vi "DeleteSubscriber.vi"(8 "ErrorIn":errorcluster, 9 "TraceQueue":refnum<queue>, 11 "TAFTraceWindowIn":refnum<class "TAFTraceWindow.lvclass">) -> (0 "ErrorOut":errorcluster, 3 "TAFTraceWindowOut":refnum<class "TAFTraceWindow.lvclass">)   [LabVIEW 2021, in "TAFTraceWindow.lvclass"]
uses:
  TAFTraceWindow.lvclass
  C:/Localdata/Projects/TriekselSoft/TriekselsoftApplicationFramework/Source/.Externals/Library_YAF/YActor/YActor.lvclass
  Library_YAF/YActor/YActor.lvclass/YActor.ctl
  Library_YAF/YActor/ExeCmd_sync.vi
  Library_YAF/YActor/private/SendCommand.vi
  Library_YAF/YActor/private/WaitForReply.vi
  Library_YAF/YActor/private/CreateLocalVI.vi
  Library_YAF/YActor/private/ExeuteInlineVI.vi
  Library_YAF/YActor/private/GetRemoteVIRef.vi
  Library_YAF/YActor/private/GetNameOfVI.vi
  Library_YAF/YActor/QuickCast.vi
  Library_YAF/YActor/private/VINameProperty.vi
  Library_YAF/YActor/private/MessageCounter.vi
  Library_YAF/YActor/InlineReferencePool.vi
  Library_YAF/YActor/private/ExecuteVI.vi
  Library_YAF/YActor/YActor.lvclass
  TAFTraceWindow.lvclass/TAFTraceWindow.ctl
  C:/Localdata/Projects/TriekselSoft/TriekselsoftApplicationFramework/Source/.Externals/Library_YAF/YAFTAF/YAFTAF.lvclass
  C:/Localdata/Projects/TriekselSoft/TriekselsoftApplicationFramework/Source/.Externals/Interface_UserInterface_IFrontPanel/IFrontPanel/IFrontPanel.lvclass
  C:/Localdata/Projects/TriekselSoft/TriekselsoftApplicationFramework/Source/IInterface/IInterface.lvclass
  C:/Localdata/Projects/TriekselSoft/TriekselsoftApplicationFramework/Source/.Externals/Interface_Object_ICreateDestroy/ICreateDestroy/ICreateDestroy.lvclass
  C:/Localdata/Projects/TriekselSoft/TriekselsoftApplicationFramework/Source/.Externals/Interface_Object_IPersistentData/IPersistentData/IPersistentData.lvclass
  C:/Localdata/Projects/TriekselSoft/TriekselsoftApplicationFramework/Source/.Externals/Interface_TAF_ITAFObject/ITAFObject/ITAFObject.lvclass
  C:/Localdata/Projects/TriekselSoft/TriekselsoftApplicationFramework/Source/.Externals/Library_TAF_TraceWindow/TAFTraceWindow/TAFTraceWindow.lvclass
  C:/Localdata/Projects/TriekselSoft/TriekselsoftApplicationFramework/Source/.Externals/INewOpenCVMat/INewOpenCVMat.lvclass
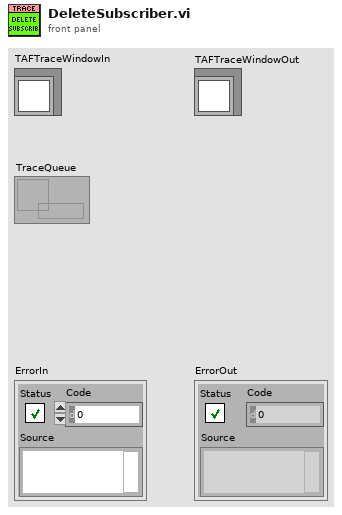
[diagram p1: front panel]
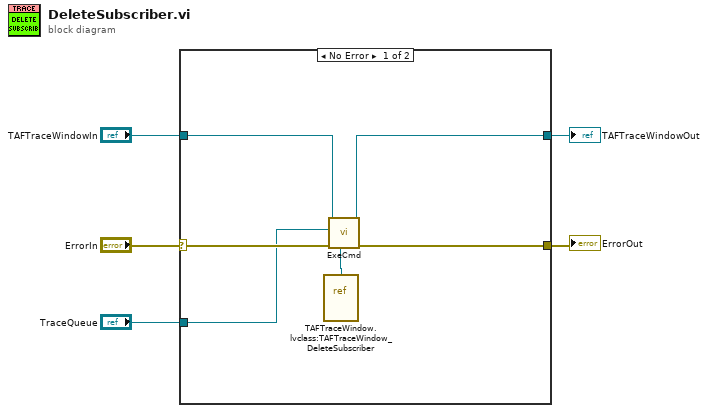
[diagram p0: block diagram]
diagram:
  n1 = case shown="No Error" "ErrorIn" {
    selector: "ErrorIn" -> [w11 w13]
    tunnel: [w6 w13] -> w4
    tunnel: [w8 w12] -> w2
    tunnel: "TAFTraceWindowIn" -> [w9 w12]
    tunnel: "TraceQueue" -> [w7 _]
    frame No Error {
      n2 = vi-ref "TAFTraceWindow.lvclass:TAFTraceWindow_DeleteSubscriber.vi"() -> (w10:refnum<vi>)
      n3 = call-poly "ExeCmd.vi"("CmdVIRef"=w10, "ErrorIn"=w11, "CmdData"=w7, "YActorIn"=w9) -> ("ErrorOut"=w6:errorcluster, "YActorOut"=w8:refnum<class "TAFTraceWindow.lvclass">)  [unwired: 5 in, 1 out]
    }
    frame Error {
    }
  }
  "ErrorOut" <- w4
  "TAFTraceWindowOut" <- w2
